vi "PhoenixVisionCom.vi"() -> ()   [LabVIEW 2018]
uses:
  Vision_class/Old vision/Controls/AI Input.ctl
  Vision_class/Old vision/Controls/AI Robot.ctl
  Vision_class/Old vision/Controls/Functions Enum.ctl
  Vision_class/Old vision/Controls/AttackerStates.ctl
  Vision_class/Old vision/Controls/PathDests.ctl
  Vision_class/Old vision/Controls/PathDest.ctl
  Vision_class/Old vision/Controls/AI Ball.ctl
  Vision_class/Old vision/Controls/Field Size.ctl
  Vision_class/Old vision/Controls/AI Judge.ctl
  Vision_class/Old vision/Controls/Command Enum.ctl
  Vision_class/Old vision/Controls/Events.ctl
  Ball_class/Ball.lvclass
  Ally_class/Ally.lvclass
  C:/Users/nicolas.oliveira/roboime/SSL_AI/Team_class/Team.lvclass
  Field_class/Field.lvclass
  Vision_class/Old vision/Controls/Estimadores.ctl
  Vision_class/Old vision/Decode SSL and Refree Wrapper Package Folder/SSL Referee Game Status.ctl
  Vision_class/Old vision/Draw Field Folder/DrawTargets.ctl
  Vision_class/Old vision/Controls/SSL Field State.ctl
  Vision_class/Old vision/Controls/SSL Detection Frame.ctl
  Vision_class/Old vision/Controls/SSL Detection Robot.ctl
  <vilib>/Analysis/Matrix/Datatypes/RealMatrix.ctl
  Vision_class/Old vision/Controls/SSL Detection Ball.ctl
  Communication_class/Communication.lvclass
  Controls/ComUDP.ctl
  Controls/ComSerial.ctl
  Controls/ComSOS.ctl
  Controls/vision_control.ctl
  Vision_class/Vision.lvclass
  Game_class/Game.lvclass
  Game_class/Game.lvclass/Game.ctl
  Team_class/Team.lvclass/Team.ctl
  Object_class/Object.lvclass/Object.ctl
  Robot_class/Robot.lvclass/Robot.ctl
  Game_class/Read AllyRef.vi
  Game_class/Read EnemyRef.vi
  Team_class/Read RobotRef.vi
  Object_class/Read x.vi
  Object_class/Read y.vi
  Robot_class/Read orientation.vi
  Robot_class/Read id.vi
  Game_class/Read FieldRef.vi
  Game_class/Read BallRef.vi
  Enemy_class/Enemy.lvclass
  Robot_class/Robot.lvclass
  C:/Users/nicolas.oliveira/roboime/SSL_AI/Object_class/Object.lvclass
  <vilib>/Analysis/Matrix/NI_Matrix.lvlib
panel:
  in  "SSL UDP RX":T1={"Local IP:"="", "Port"=10006, "Server IP:"="224.5.23.2"}
  in  "RefBox UDP RX":T1={"Local IP:"="", "Port"=10003, "Server IP:"="224.5.23.1"}
  in  "Com SOS":T2={"UDP SOS TX "=FALSE, "SOS Port: 2"=10025, "SOS Port: "=10021, "SOS Address:"="192.168.0.101"}
  in  "Com Serial":T3
  in  "Com UDP":T4={"UDP GrSim TX"=TRUE, "Address:"="127.0.0.1", "Port:"=20011}
  in  "Communication in":refnum<class "Communication.lvclass">
  out "FPS Com":dbl
  in  "Frame and Field Size out Ref":T5 {"Detection Frame Out"."robots_blue"."height" format="%+4.3f"; "Detection Frame Out"."robots_blue"."pixel_y" format="%+4.3f"; "Detection Frame Out"."robots_blue"."pixel_x" format="%+4.3f"; "Detection Frame Out"."robots_blue"."orientation" format="%+4.3f"; "Detection Frame Out"."robots_blue"."y" format="%+4.3f"; "Detection Frame Out"."robots_blue"."confidence" format="%4.3f"; "Detection Frame Out"."robots_blue"."x" format="%+4.3f"; "Detection Frame Out"."robots_yellow"."height" format="%+4.3f"; "Detection Frame Out"."robots_yellow"."pixel_y" format="%+4.3f"; "Detection Frame Out"."robots_yellow"."pixel_x" format="%+4.3f"; "Detection Frame Out"."robots_yellow"."orientation" format="%+4.3f"; "Detection Frame Out"."robots_yellow"."y" format="%+4.3f"; "Detection Frame Out"."robots_yellow"."confidence" format="%4.3f"; "Detection Frame Out"."robots_yellow"."x" format="%+4.3f"}
  in  "Draw Targets?":T10={"Attacker"=TRUE, "Striker"=TRUE, "Goalie"=TRUE, "Defender"=TRUE, "kick"=TRUE, "Est Ball"=TRUE, "Est Robot"=FALSE, "Path S"=FALSE, "Path C"=FALSE, "Dngr.Enemy"=TRUE, "2nd Striker"=TRUE}
  out "2D Picture":picture
  in  "Draw Field":bool=TRUE
  out "FPS Draw Field":dbl
  out "FPS test":dbl
  out "x":dbl
  out "y":dbl
  out "orientation":dbl
  out "id":i32
  in  "Index":i32
  out "size ally":i32
  out "x 2":dbl
  out "y 2":dbl
  out "orientation 2":dbl
  out "id 2":i32
  in  "Index 2":i32
  out "size(s) enemy":i32
  in  "SSL Referee Game Status Ref":T11 {"Time" format="%<%.3X %x>T"; "Blue Timeout Remaining" format="%<%M:%S>t"; "Yellow Timeout Remaining" format="%<%M:%S>t"; "Time Left" format="%<%M:%S>t"}
  out "GUI Game Status":T11 {"Time" format="%<%.3X %x>T"; "Blue Timeout Remaining" format="%<%M:%S>t"; "Yellow Timeout Remaining" format="%<%M:%S>t"; "Time Left" format="%<%M:%S>t"}
  out "SSL Referee Game Status":T11 {"Time" format="%<%.3X %x>T"; "Blue Timeout Remaining" format="%<%M:%S>t"; "Yellow Timeout Remaining" format="%<%M:%S>t"; "Time Left" format="%<%M:%S>t"}
  out "FPS referee":dbl
  in  "Command":string(combo)="Auto"
  in  "Goalie":string(combo)="0"
  out "RX":bool
  in  "Estimador":T12=enum."Kalman"
  in  "ignora lado?":bool
  in  "ignora esquerda?":bool
  in  "Side":enum16{"Esquerdo", "Direito"}(ring) caption="Enum"
  in  "Team":enum16{"Azul", "Amarelo"}(ring) caption="Enum"
  out "FieldRef":refnum<class "Field.lvclass">
  out "AllyRef":refnum<class "Ally.lvclass">
  out "BallRef":refnum<class "Ball.lvclass">
  in  "Defense width":i32=1000
  in  "Defense stretch":i32=2000
  out "AI State":T13={"our_robots"=[], "enemy_robots"=[], "balls"=[], "geometry"={"line_width"=0, "field_length"=0, "field_width"=0, "boundary_width"=0, "referee_width"=0, "goal_width"=0, "goal_depth"=0, "goal_wall_width"=0, "center_circle_radius"=0, "defense_radius"=0, "defense_stretch"=0, "free_kick_from_defense_dist"=0, "penalty_spot_from_field_line_dist"=0, "penalty_line_from_spot_dist"=0}, "IA Judge"={"stage"="", "command"="", "our_goalie_id"=0.0, "enemy_goalie_id"=0.0, "command enum"=enum."Halt", "Time"=enum."Azul"}, "Received Timestamp"=timestamp(0 s since 1904-01-01), "Events"={"Touch"=FALSE, "Ball out"=FALSE, "id touch"=0.0, "Ball out of \nVision"=FALSE, "Ball inside \nGoalie area"=FALSE, "Robot not responding"=FALSE, "Robots responding status"=[1.0, 1.0, 1.0, 1.0, 1.0, 1.0], "Enemy Ball \nPossession"=FALSE, "Pass State"=FALSE, "id end of pass"=0.0, "Kick"=FALSE, "Id ini Possession"=0.0, "Ball Possesion"=FALSE, "Id Possesion"=0.0, "Direct Kick"=FALSE, "2nd Strk Ativo"=FALSE}}
  out "FPS vision":dbl
  in  "Id camera\nsup esq":dbl
  in  "Id camera\ninf esq":dbl=1.0
  in  "Id camera\nsup dir":dbl=3.0
  in  "Id camera\ninf dir":dbl=2.0
  # "left goal"
  # "right goal"
  # "vision computer"
  # "Score"
  # "Red Cards"
  # "Yellow Cards"
  # "Timeouts Left"
  # "Timeout Remaining"
  # "Goalie ID"
  # "Score"
  # "Red Cards"
  # "Yellow Cards"
  # "Timeouts Left"
  # "Timeout Remaining"
  # "Goalie ID"
  # "Score"
  # "Red Cards"
  # "Yellow Cards"
  # "Timeouts Left"
  # "Timeout Remaining"
  # "Goalie ID"
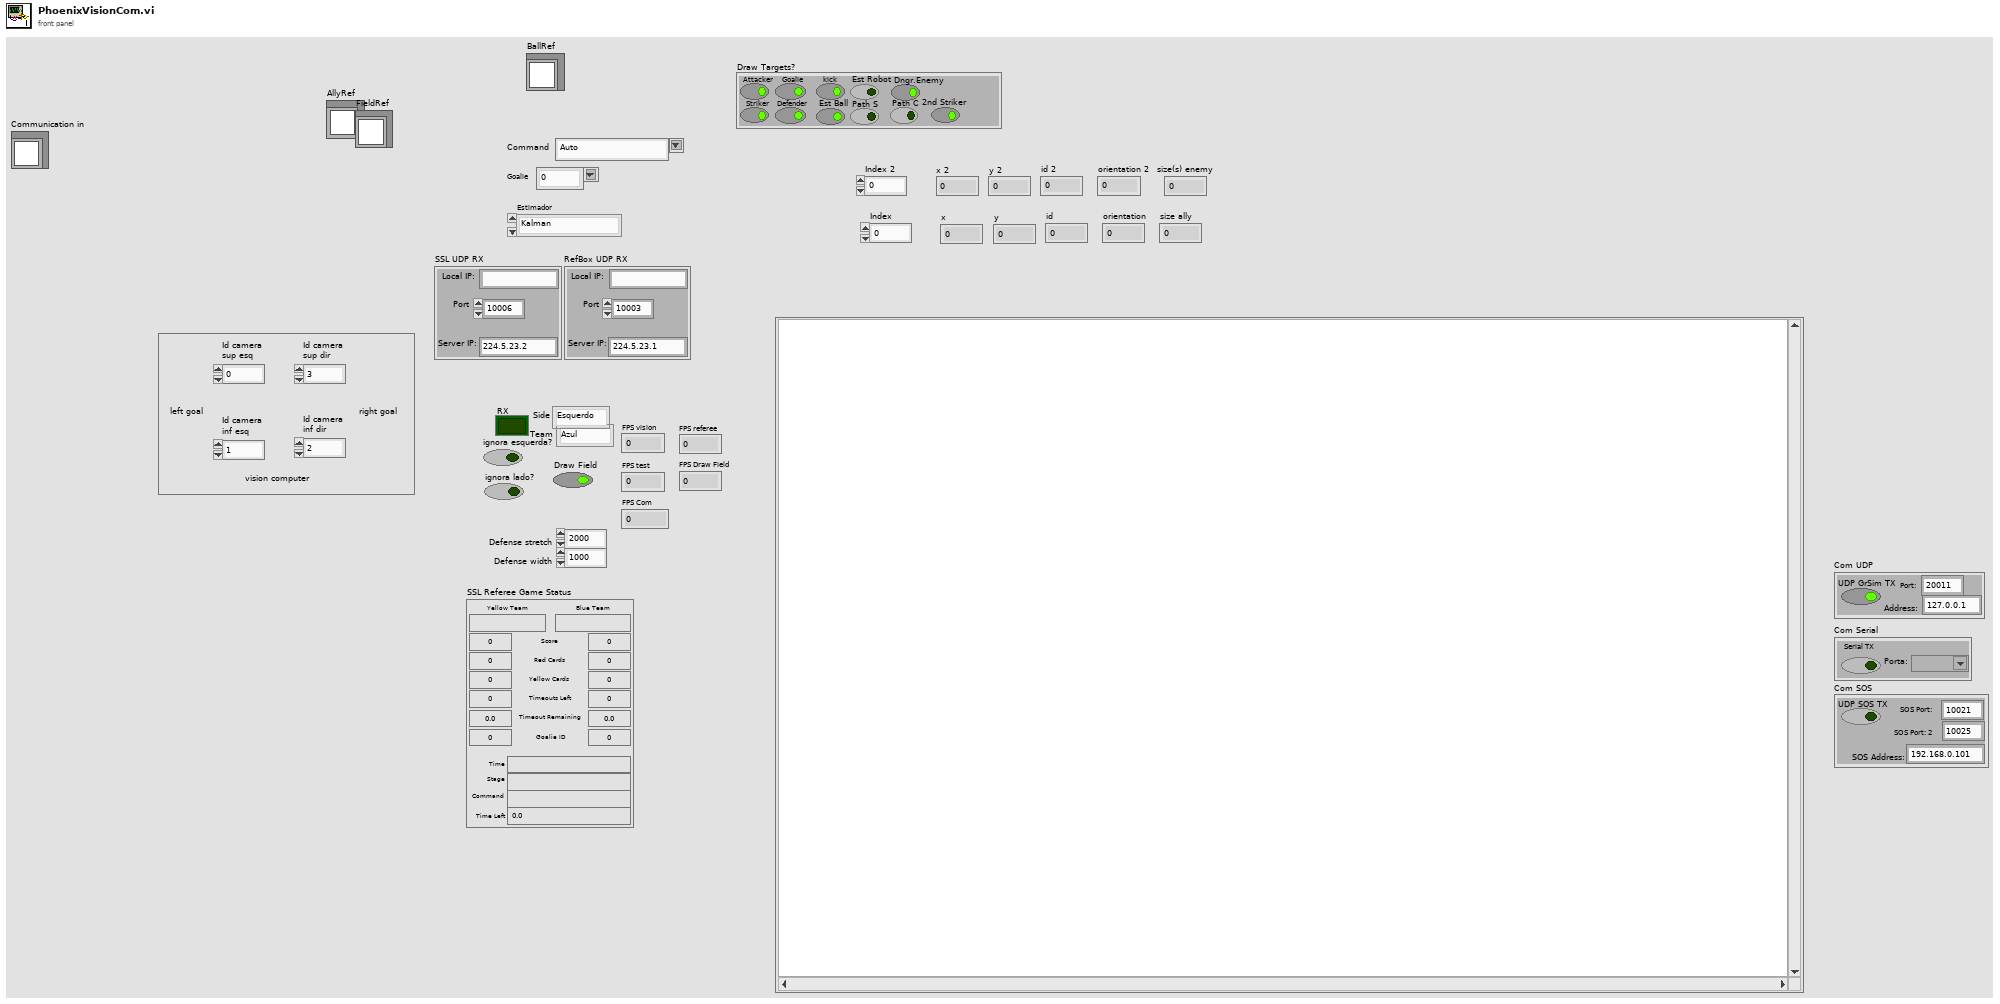
[diagram p1: front panel]
types:
  T1 = typedef "vision_control.ctl" = cluster{"Local IP:":string, "Port":i32, "Server IP:":string}
  T2 = typedef "ComSOS.ctl" = cluster{"UDP SOS TX ":bool, "SOS Port: 2":u16, "SOS Port: ":u16, "SOS Address:":string}
  T3 = typedef "ComSerial.ctl" = cluster{"Serial TX":bool, "Porta:":refnum<visa-resource-name>}
  T4 = typedef "ComUDP.ctl" = cluster{"UDP GrSim TX":bool, "Address:":string, "Port:":u16}
  T5 = typedef "SSL Field State.ctl" = cluster{"Detection Frame Out":T6, "Field Size Out":cluster{"line_width":u32, "field_length":u32, "field_width":u32, "boundary_width":u32, "referee_width":u32, "goal_width":u32, "goal_depth":u32, "goal_wall_width":u32, "center_circle_radius":u32, "defense_radius":u32, "defense_stretch":u32, "free_kick_from_defense_dist":u32, "penalty_spot_from_field_line_dist":u32, "penalty_line_from_spot_dist":u32}, "Received Time Stamp":timestamp}
  T6 = typedef "SSL Detection Frame.ctl" = cluster{"frame_number":u32, "t_capture":dbl, "t_sent":dbl, "camera_id":u32, "robots_yellow":T7[], "robots_blue":T7[], "balls":T9[], "Valid":bool, "Time Stamp":timestamp}
  T7 = typedef "SSL Detection Robot.ctl" = cluster{"x":sgl, "robot_id":u32, "confidence":sgl, "y":sgl, "orientation":sgl, "pixel_x":sgl, "pixel_y":sgl, "height":sgl, "Valid":bool, "Time Stamp":timestamp, "x_k|k":T8, "Pk|k":T8, "Previous Time Stamp":timestamp, "R":T8}
  T8 = typedef "NI_Matrix.lvlib/RealMatrix.ctl" = dbl[][]
  T9 = typedef "SSL Detection Ball.ctl" = cluster{"x":sgl, "area":u32, "confidence":sgl, "y":sgl, "z":sgl, "pixel_x":sgl, "pixel_y":sgl, "Valid":bool, "Time Stamp":timestamp, "x_k|k":T8, "Pk|k":T8, "Id":u32, "Previous Time Stamp":timestamp, "R":T8}
  T10 = typedef "DrawTargets.ctl" = cluster{"Attacker":bool, "Striker":bool, "Goalie":bool, "Defender":bool, "kick":bool, "Est Ball":bool, "Est Robot":bool, "Path S":bool, "Path C":bool, "Dngr.Enemy":bool, "2nd Striker":bool}
  T11 = typedef "SSL Referee Game Status.ctl" = cluster{"Stage":string, "Command":string, "Time Left":dbl, "Yellow Team":string, "Blue Team":string, "Yellow Score":u32, "Blue Score":u32, "Yellow Red Cards":u32, "Blue Red Cards":u32, "Yellow Yellow Cards":u32, "Blue Yellow Cards":u32, "Yellow Timeouts Left":u32, "Blue Timeouts Left":u32, "Yellow Timeout Remaining":dbl, "Blue Timeout Remaining":dbl, "Yellow Goalie Id":u32, "Blue Goalie Id":u32, "Time":timestamp}
  T12 = typedef "Estimadores.ctl" = enum16{"Nenhum", "Simples", "Kalman"}
  T13 = typedef "AI Input.ctl" = cluster{"our_robots":T14[], "enemy_robots":T14[], "balls":T19[], "geometry":T20, "IA Judge":T21, "Received Timestamp":timestamp, "Events":T23}
  T14 = typedef "AI Robot.ctl" = cluster{"id":u32, "function":T15, "x":dbl, "y":dbl, "orientation":dbl, "v_tangent":dbl, "v_normal":dbl, "v_ang":dbl, "kick_x":dbl, "kick_z":dbl, "dribble":bool, "Timestamp":timestamp, "estimatives":cluster{"est_v_tangent":dbl, "est_v_normal":dbl, "est_vx":dbl, "est_vy":dbl, "Pos Robot Est":dbl[]}, "dest_x_kick":dbl, "dest_y_kick":dbl, "Gap Coord":dbl[], "States":T16, "Path ":dbl[][], "Path  Smooth":dbl[][], "Dest":T17}
  T15 = typedef "Functions Enum.ctl" = enum16{"2nd Striker", "Attacker", "Goalie", "Defender", "Striker", "Goto 0", "Dummy", "Kicker", "ZigZag 0", "ZigZag 1", "ZigZag 2", "ZigZag 3", "ZigZag 4", "ZigZag 5", "ZigZag 6", "ZigZag 7", "ZigZag 8", ""}
  T16 = typedef "AttackerStates.ctl" = enum16{"Pass", "GoToTangent", "BallGetting", "GoToKick", ""}
  T17 = typedef "PathDests.ctl" = T18[]
  T18 = typedef "PathDest.ctl" = cluster{"dest_x":dbl, "dest_y":dbl, "dest_orientation":dbl, "dest_vel":dbl}
  T19 = typedef "AI Ball.ctl" = cluster{"x":dbl, "y":dbl, "timestamp":timestamp, "Vel_x":dbl, "Vel_y":dbl, "Pos Bola Est":dbl[]}
  T20 = typedef "Field Size.ctl" = cluster{"line_width":u32, "field_length":u32, "field_width":u32, "boundary_width":u32, "referee_width":u32, "goal_width":u32, "goal_depth":u32, "goal_wall_width":u32, "center_circle_radius":u32, "defense_radius":u32, "defense_stretch":u32, "free_kick_from_defense_dist":u32, "penalty_spot_from_field_line_dist":u32, "penalty_line_from_spot_dist":u32}
  T21 = typedef "AI Judge.ctl" = cluster{"stage":string, "command":string, "our_goalie_id":dbl, "enemy_goalie_id":dbl, "command enum":T22, "Time":enum16{"Azul", "Amarelo"}}
  T22 = typedef "Command Enum.ctl" = enum16{"Halt", "Stop", "Force Start", "PKA Normal Start", "Prepare Kickoff Ally", "PKE Normal Start", "Prepare Kickoff Enemy", "Prepare Penalty Ally", "PPA Normal Start", "Prepare Penalty Enemy", "PPE Normal Start", "Direct Free Enemy", "Direct Free Ally", "Indirect Free Enemy", "Indirect Free Ally", "Timeout Enemy", "Timeout Ally", "Goal Enemy", "Goal Ally", "Ball Placement Enemy", "Ball Placement Ally", "Normal Half Time", "Extra Time Break", "Extra Half Time", "None", "Post Game"}
  T23 = typedef "Events.ctl" = cluster{"Touch":bool, "Ball out":bool, "id touch":dbl, "Ball out of \nVision":bool, "Ball inside \nGoalie area":bool, "Robot not responding":bool, "Robots responding status":dbl[], "Enemy Ball \nPossession":bool, "Pass State":bool, "id end of pass":dbl, "Kick":bool, "Id ini Possession":dbl, "Ball Possesion":bool, "Id Possesion":dbl, "Direct Kick":bool, "2nd Strk Ativo":bool}
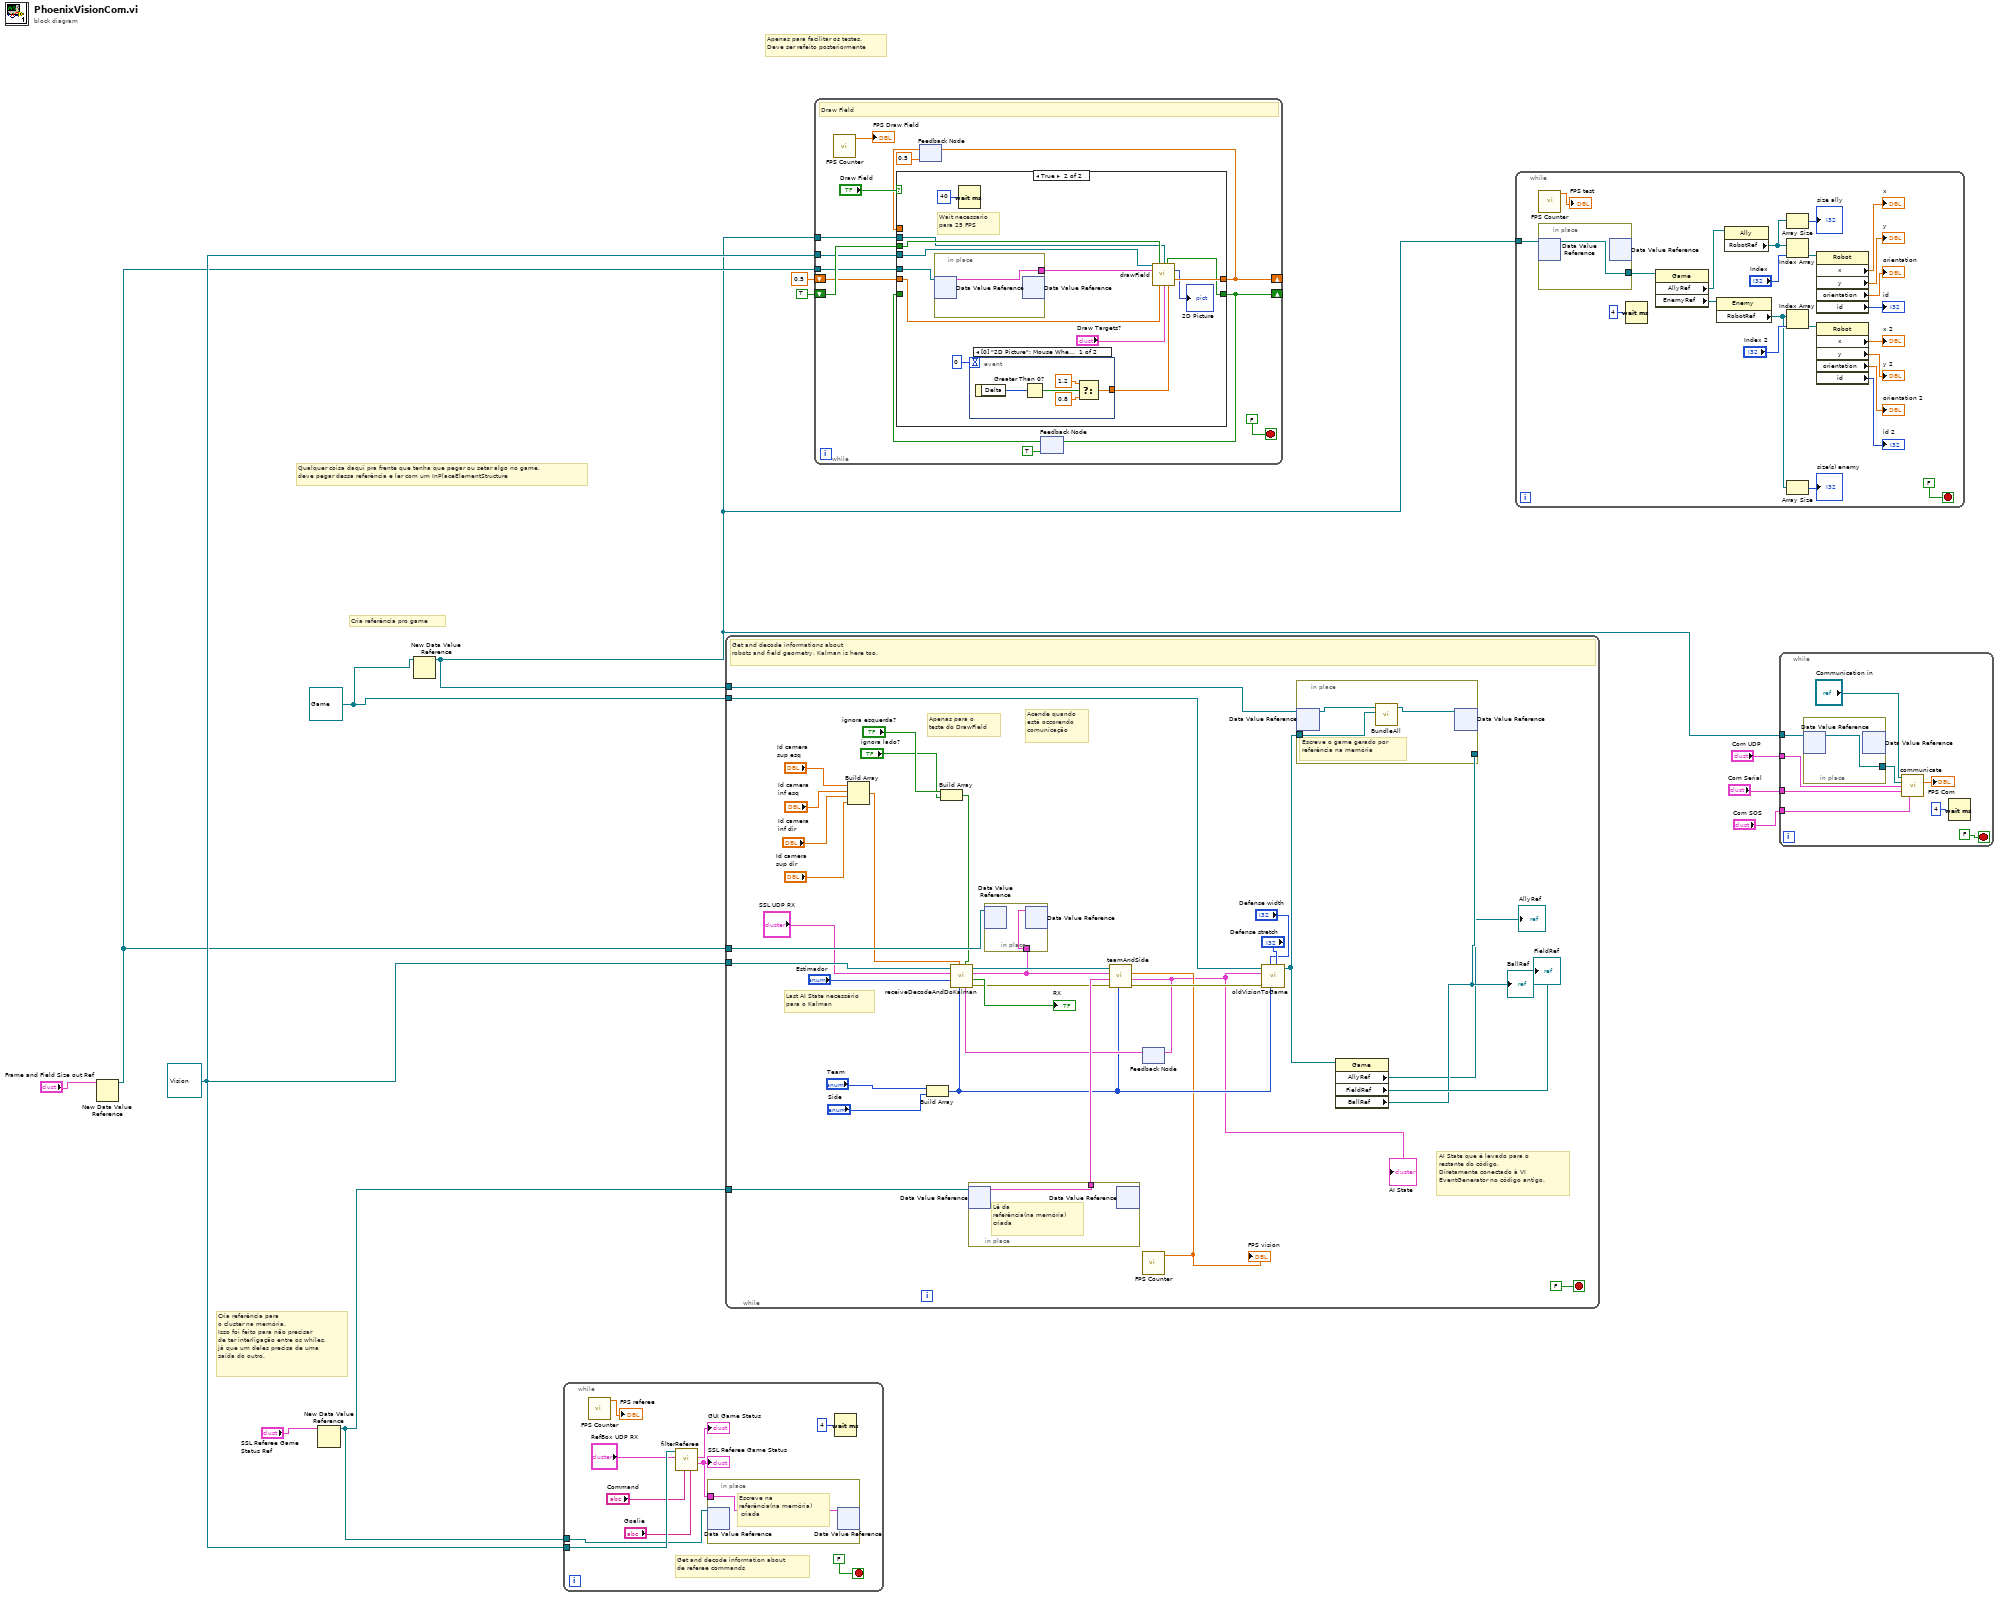
[diagram p0: block diagram]
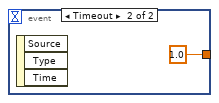
[diagram p3: hidden frame]
diagram:
  w5 = refnum<class "Game.lvclass"> refnum ("Game")
  w8 = refnum<class "Vision.lvclass"> refnum ("Vision")
  # "Apenas para facilitar os testes.\nDeve ser refeito posteriormente"
  # "Qualquer coisa daqui pra frente que tenha que pegar ou setar algo no game,\ndeve pegar dessa referência e ler com um InPlaceElementStructure"
  # "Cria referência pro game"
  # "Cria referência para\no cluster na memória.\nIsso foi feito para não precisar\nde ter interligação entre os whiles,\njá que um deles precisa de uma\nsaída do outro."
  n1 = New Data Value Reference(data value="Frame and Field Size out Ref") -> (data value reference=w6:refnum<data-value>)  [unwired: 1 in, 1 out]
  n2 = New Data Value Reference(data value="SSL Referee Game Status Ref") -> (data value reference=w11:refnum<data-value>)  [unwired: 1 in, 1 out]
  n3 = New Data Value Reference(data value=w5) -> (data value reference=w4:refnum<data-value>)  [unwired: 1 in, 1 out]
  n4 = while {
    tunnel: w8 -> [w21]
    tunnel: w11 -> [w19]
    stop <- FALSE stop-if-true
    # "Get and decode information about\nde referee commands"
    n5 = call "FPS Counter.vi"() -> ("Numeric"=→"FPS referee":dbl)  [unwired: 11 in]
    n6 = call "filterReferee.vi"("Goleiro"="Goalie", "Command"="Command", "RefBox UDP RX"="RefBox UDP RX", "Vision in"=w21) -> ("SSL Referee Game Status"=w18:T11, "GUI Game Status"=→"GUI Game Status":T11)  [unwired: 4 in, 2 out]
    "SSL Referee Game Status" <- w18
    n7 = in-place {
      in-place-border: w18 -> [w23]
      # "Escreve na\nreferência(na memória)\n criada"
      n8 = in-place-dvr #1(w19) -> ()  [unwired: 2 out]
      n9 = in-place-dvr #1(w23) -> ()  [unwired: 2 out]
    }
    n10 = Wait (ms)(milliseconds to wait=u32 4) -> ()  [unwired: 1 out]
  }
  n11 = while {
    tunnel: w8 -> [w53]
    tunnel: w11 -> [w51]
    tunnel: w4 -> [w50]
    tunnel: w6 -> [w38]
    tunnel: w5 -> [w36]
    stop <- FALSE stop-if-true
    # "Apenas para o\nteste do DrawField"
    # "Acende quando\nestá occorendo\ncomunicação"
    # "Last AI State necessário\npara o Kalman"
    # "AI State que é levado para o\nrestante do código.\nDiretamente conectado à VI\nEventGenerator no código antigo."
    # "Get and decode informations about\nrobots and field geometry. Kalman is here too."
    n12 = Build Array("Id camera\nsup esq", "Id camera\ninf esq", "Id camera\ninf dir", "Id camera\nsup dir") -> (w27:dbl[])
    n13 = Build Array("Team", "Side") -> (w42:u16[])
    n14 = Build Array("ignora esquerda?", "ignora lado?") -> (w30:bool[])
    n15 = in-place {
      in-place-border: [w62] -> w52
      # "Lê da\nreferência(na memória)\ncriada"
      n16 = in-place-dvr #2(w51) -> (w62:T11)  [unwired: 1 out]
      n17 = in-place-dvr #2() -> ()  [unwired: 1 in, 2 out]
    }
    n18 = feedback #3() -> (w45:T13)  [unwired: 1 in]
    n19 = call "receiveDecodeAndDoKalman.vi"("Last AI State"=w45, "ignora ?"=w30, "team/side"=w42, "cameras array"=w27, "Estimador"="Estimador", "SSL UDP RX"="SSL UDP RX", "Vision in"=w53) -> ("error out"=w44:errorcluster, "RX"=→"RX":bool, "Frame and Field Size out"=w37:T5, "Vision out"=w41:refnum<class "Vision.lvclass">)  [unwired: 1 in]
    n20 = in-place {
      in-place-border: w37 -> [w58]
      n21 = in-place-dvr #4(w38) -> ()  [unwired: 2 out]
      n22 = in-place-dvr #4(w58) -> ()  [unwired: 2 out]
    }
    n23 = call "FPS Counter.vi"() -> ("Numeric"=w40:dbl)  [unwired: 11 in]
    "FPS vision" <- w40
    n24 = call "teamAndSide.vi"("Comm RX FPS"=w40, "team/side"=w42, "error in (no error)"=w44, "Game Status"=w52, "Field State Input"=w37, "Vision in"=w41) -> ("error out"=w43:errorcluster, "IA State"=w39:T13)  [unwired: 3 in, 1 out]
    "AI State" <- w39
    n25 = feedback-in #3(w39) -> ()
    n26 = call "oldVisionToGame.vi"("Defense stretch"="Defense stretch", "Team/ Side"=w42, "Defense width"="Defense width", "error in (no error)"=w43, "IA State"=w39, "Game in"=w36) -> ("Game out"=w48:refnum<class "Game.lvclass">)  [unwired: 4 in, 1 out]
    n27 = property class="Game"(reference=w48) -> ("AllyRef"=→"AllyRef":refnum<class "Ally.lvclass">, "FieldRef"=→"FieldRef":refnum<class "Field.lvclass">, "BallRef"=w49:refnum<class "Ball.lvclass">)  [unwired: 1 in, 2 out]
    "BallRef" <- w49
    n28 = in-place {
      in-place-border: w49 -> [_]
      in-place-border: w48 -> [w60]
      # "Escreve o game gerado por\nreferência na memória"
      n29 = in-place-dvr #5(w50) -> (w61:refnum<class "Game.lvclass">)  [unwired: 1 out]
      n30 = call "BundleAll.vi"("Game in\natualized"=w60, "Game in"=w61) -> ("Game out"=w59:refnum<class "Game.lvclass">)  [unwired: 8 in, 1 out]
      n31 = in-place-dvr #5(w59) -> ()  [unwired: 2 out]
    }
  }
  n32 = while {
    shift-right: [w68] -> _
    shift-left: 0.5 ("New Scale") -> [w75]
    shift-right: [w70] -> _
    shift-left: TRUE ("AutoScale Out") -> [w76]
    tunnel: w8 -> [w74]
    tunnel: w4 -> [w73]
    tunnel: w6 -> [w72]
    stop <- FALSE stop-if-true
    # "Draw Field"
    n33 = call "FPS Counter.vi"() -> ("Numeric"=→"FPS Draw Field":dbl)  [unwired: 11 in]
    n34 = feedback #6(0.5 ("New Scale")) -> (w67:dbl)
    n35 = feedback #7(TRUE ("AutoScale Out")) -> (w69:bool)
    n36 = case shown="True" "Draw Field" {
      tunnel: [w77 w91] -> w68
      tunnel: [w78 w90] -> w70
      tunnel: w76 -> [_ w89]
      tunnel: w75 -> [_ w87]
      tunnel: w74 -> [_ w82]
      tunnel: w73 -> [_ w81]
      tunnel: w72 -> [_ w80]
      tunnel: w69 -> [w78 _]
      tunnel: w67 -> [w77 _]
      frame False {
      }
      frame True {
        # "Wait necessario\npara 25 FPS"
        n37 = in-place {
          in-place-border: [w92] -> w79
          n38 = in-place-dvr #8(w80) -> (w92:T5)  [unwired: 1 out]
          n39 = in-place-dvr #8() -> ()  [unwired: 1 in, 2 out]
        }
        n40 = Wait (ms)(milliseconds to wait=u32 40) -> ()  [unwired: 1 out]
        n41 = event shown="[0] \"2D Picture\": Mouse Wheel" {
          selector: _ -> [_ _]
          dyn-events: _ -> [_ _]
          timeout: 0 -> [_ _]
          tunnel: [w93 1.0] -> w84
          event "2D Picture": Mouse Wheel {
            n42 = event-data() -> ("Delta"=w97:i32)  [unwired: 1 in]
            n43 = Greater Than 0?(x=w97) -> (x > 0?=w96:bool)
            n44 = Select(t=1.2, s=w96, f=0.8) -> (s? t:f=w93:dbl)
          }
          event Timeout {
            n45 = event-data() -> ()  [unwired: 1 in, 3 out]
          }
        }
        n46 = call "drawField.vi"("Vision in"=w82, "AutoScale"=w89, "Game reference"=w81, "Field State Input"=w79, "Scale mm/pixel"=w87, "Draw Targets?"="Draw Targets?", "Zoom"=w84) -> ("AutoScale Out"=w90:bool, "2D Picture"=→"2D Picture":picture, "Scale Out"=w91:dbl)  [unwired: 4 in, 2 out]
      }
    }
    n47 = feedback-in #6(w68) -> ()
    n48 = feedback-in #7(w70) -> ()
  }
  n49 = while {
    tunnel: w4 -> [w120]
    stop <- FALSE stop-if-true
    n50 = call "FPS Counter.vi"() -> ("Numeric"=→"FPS test":dbl)  [unwired: 11 in]
    n51 = in-place {
      in-place-border: [w122] -> w119
      n52 = in-place-dvr #9(w120) -> (w122:refnum<class "Game.lvclass">)  [unwired: 1 out]
      n53 = in-place-dvr #9() -> ()  [unwired: 1 in, 2 out]
    }
    n54 = Wait (ms)(milliseconds to wait=u32 4) -> ()  [unwired: 1 out]
    n55 = property class="Game"(reference=w119) -> ("AllyRef"=w116:refnum<class "Ally.lvclass">, "EnemyRef"=w99:refnum<class "Enemy.lvclass">)  [unwired: 1 in, 2 out]
    n56 = property class="Enemy"(reference=w99) -> ("RobotRef"=w101:refnum<class "Robot.lvclass">[])  [unwired: 1 in, 2 out]
    n57 = property class="Ally"(reference=w116) -> ("RobotRef"=w109:refnum<class "Robot.lvclass">[])  [unwired: 1 in, 2 out]
    n58 = Array Size(array=w109) -> (size(s)=→"size ally":i32)
    n59 = Index Array(array=w109, index="Index") -> (element=w115:refnum<class "Robot.lvclass">)
    n60 = Index Array(array=w101, index="Index 2") -> (element=w107:refnum<class "Robot.lvclass">)
    n61 = Array Size(array=w101) -> (size(s)=→"size(s) enemy":i32)
    n62 = property class="Robot"(reference=w115) -> ("x"=→"x":dbl, "y"=→"y":dbl, "orientation"=→"orientation":dbl, "id"=→"id":i32)  [unwired: 1 in, 2 out]
    n63 = property class="Robot"(reference=w107) -> ("x"=→"x 2":dbl, "y"=→"y 2":dbl, "orientation"=→"orientation 2":dbl, "id"=→"id 2":i32)  [unwired: 1 in, 2 out]
  }
  n64 = while {
    tunnel: w4 -> [w131]
    tunnel: "Com UDP" -> [w125]
    tunnel: "Com Serial" -> [w124]
    tunnel: "Com SOS" -> [w123]
    stop <- FALSE stop-if-true
    n65 = in-place {
      in-place-border: [w132] -> w130
      n66 = in-place-dvr #10(w131) -> (w132:refnum<class "Game.lvclass">)  [unwired: 1 out]
      n67 = in-place-dvr #10() -> ()  [unwired: 1 in, 2 out]
    }
    n68 = call-dynamic "communicate.vi"("Communication in"="Communication in", "Game"=w130, "Com UDP"=w125, "Com Serial"=w124, "Com SOS"=w123) -> ("Comm TX FPS"=→"FPS Com":dbl)  [unwired: 8 in, 2 out]
    n69 = Wait (ms)(milliseconds to wait=u32 4) -> ()  [unwired: 1 out]
  }
